vi "LSCI332 GetRamp.vi"(0 "VISA Rsrc":refnum<visa-resource-name>="GPIB0::12::INSTR", 5 "Boucle(1)":u32(ring) caption="Boucle" items=["Boucle 1", "Boucle 2"], 11 "error in (no error)":errorcluster) -> (4 "Paramètres de Rampe":cluster{"Rampe activée":bool, "RateVal":dbl} {"RateVal" step=0.1}, 15 "error out":errorcluster)   [LabVIEW 2019]
doc: "Ce VI lit les paramètres limites de contrôle et ceux de stabilisation du contrôleur."
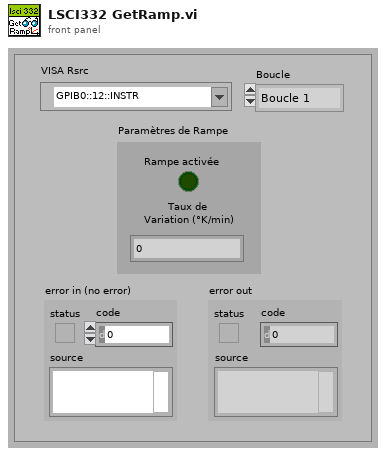
[diagram p1: front panel]
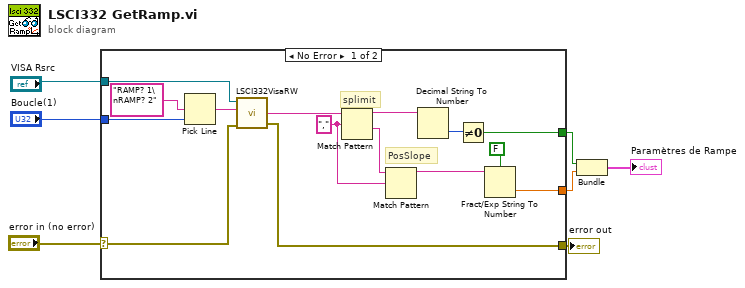
[diagram p0: block diagram]
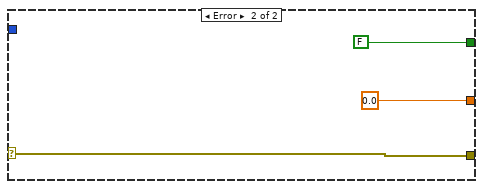
[diagram p2: hidden frame]
diagram:
  n1 = case shown="No Error" "error in (no error)" {
    selector: "error in (no error)" -> [w21 w25]
    tunnel: "VISA Rsrc" -> [w22 _]
    tunnel: "Boucle(1)" -> [w19 _]
    tunnel: [w13 w25] -> w5
    tunnel: [w12 0.0] -> w3
    tunnel: [w8 FALSE] -> w2
    frame No Error {
      w15 = "," ("regular expression")
      # "PosSlope"
      # "splimit"
      n2 = Pick Line(multi-line string="RAMP? 1\nRAMP? 2", line index=w19) -> (output string=w18:string)  [unwired: 1 in]
      n3 = call <userlib>:"LSCI332VisaRW.vi"("error in (no error)"=w21, "ChaineCom"=w18, "VISA Rsrc"=w22) -> ("error out"=w13:errorcluster, "ChaineRep"=w17:string)  [unwired: 4 in, 2 out]
      n4 = Match Pattern(string=w17, regular expression=w15) -> (before substring=w10:string, after substring=w16:string)  [unwired: 1 in, 2 out]
      n5 = Match Pattern(string=w16, regular expression=w15) -> (before substring=w14:string)  [unwired: 1 in, 3 out]
      n6 = Decimal String To Number(string=w10) -> (number=w9:i32)  [unwired: 2 in, 1 out]
      n7 = Not Equal To 0?(x=w9) -> (x != 0?=w8:bool)
      n8 = Fract/Exp String To Number(use system decimal point (T)=FALSE, string=w14) -> (number=w12:dbl)  [unwired: 2 in, 1 out]
    }
    frame Error {
    }
  }
  "error out" <- w5
  n9 = Bundle(w2, w3) -> (→"Paramètres de Rampe":cluster{bool, dbl})  [unwired: 1 in]
